vi "Cargo Arm Auto Speed.vi"(1 "Current Distance (x)":dbl) -> (0 "Final Speed":dbl)   [LabVIEW 2018]
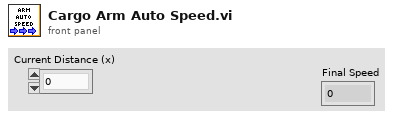
[diagram p1: front panel]
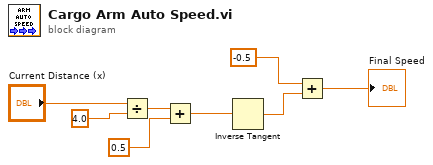
[diagram p0: block diagram]
diagram:
  n1 = Divide(x="Current Distance (x)", y=4.0) -> (x/y=w6:dbl)
  n2 = Add(x=w6, y=0.5) -> (x+y=w4:dbl)
  n3 = Inverse Tangent(1:w4) -> (0:w3:dbl)
  n4 = Add(x=-0.5, y=w3) -> (x+y=→"Final Speed":dbl)
